vi "Main1.0.vi"() -> ()   [LabVIEW 2013]
panel:
  out "Log":string
  in  "Return":bool
  in  "DataCheckOut":bool
  in  "Setup":bool
  in  "EStop":bool
  in  "显示":enum32{"参数配置", "结果显示", "帮助"}(tab)
  in  "数据帧":T1
  in  "管理帧":T2
  in  "充电帧":T3
  in  "ECALL帧":T4
  in  "任意帧":T5
  in  "终端号码1":T6
  in  "终端号码2":T7
  in  "白名单号码":T8
  in  "黑名单号码":T9
  in  "ACC唤醒":T10
  in  "休眠":bool
  in  "CAN唤醒":bool
  in  "ACC唤醒":bool
  in  "短信唤醒":bool
  in  "电话唤醒":bool
  in  "ECALL唤醒":bool
  in  "长安测试配置":bool
  in  "江淮测试配置":bool
  in  "五菱测试配置":bool
  in  "长丰测试配置":bool
  in  "海马测试配置":bool
  in  "B+电压":u16(ring) items=["5.9V", "6.5V", "9V", "12V", "16V"]
  in  "休眠电流限值":dbl
  in  "工作电流限值":dbl
  in  "循环次数":dbl
  in  "间隔时间":dbl
  out "登录时间":dbl
  out "异常次数":dbl
  out "登录结果":bool
  out "TBOX状态":bool
  out "任意帧唤醒结果":T11
  out "无效短信唤醒结果":T11
  out "黑名单电话号码唤醒结果":T11
  out "白名单电话号码唤醒结果":T11
  out "指令短信唤醒结果":T11
  out "ECALL帧唤醒结果":T11
  out "充电帧唤醒结果":T11
  out "管理帧唤醒结果":T11
  out "数据帧唤醒结果":T11
  out "ACC唤醒结果":T11
  out "ACC异常计数":dbl caption="异常计数"
  out "管理帧异常计数":dbl caption="异常计数"
  out "数据帧异常计数":dbl caption="异常计数"
  out "充电帧异常计数":dbl caption="异常计数"
  out "ECALL帧异常计数":dbl caption="异常计数"
  out "任意帧异常计数":dbl caption="异常计数"
  out "指令短信异常计数":dbl caption="异常计数"
  out "无效短信异常计数":dbl caption="异常计数"
  out "白名单异常计数":dbl caption="异常计数"
  out "黑名单异常计数":dbl caption="异常计数"
  in  "Start":bool
  # "公用参数"
  # "测试流程选择"
  # "配置文件选择"
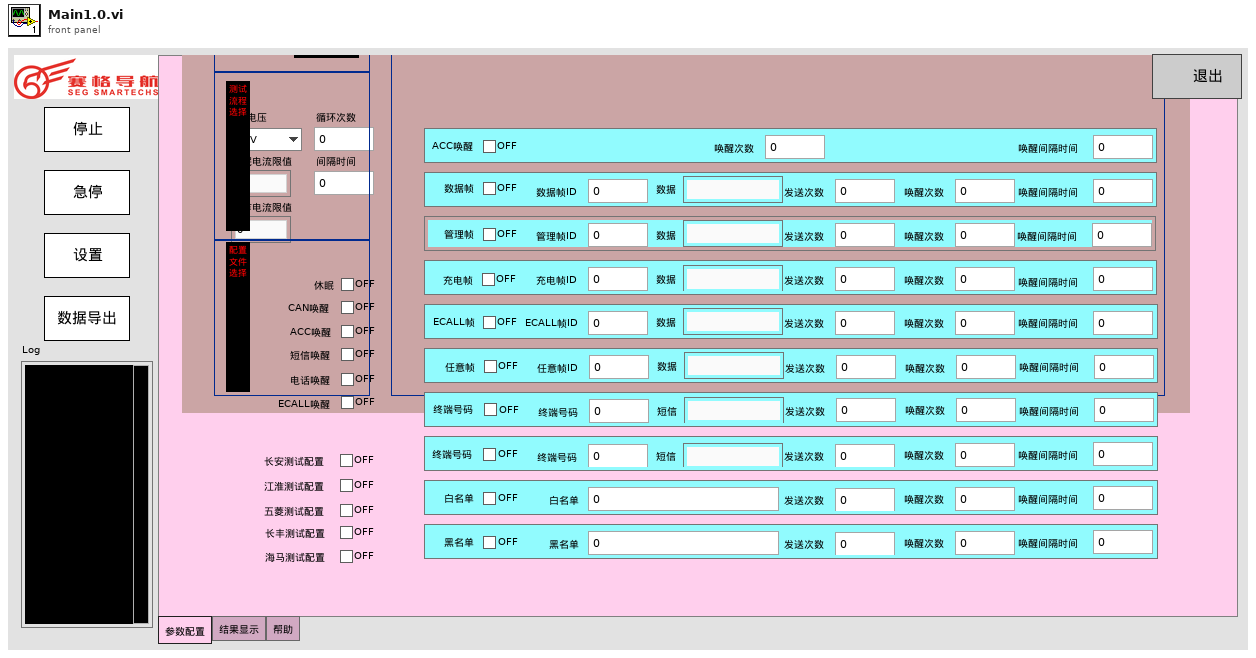
[diagram p1: front panel]
types:
  T1 = cluster{"数据帧":bool, "数据帧ID":dbl, "数据帧数据":string, "数据帧次数":dbl, "数据帧唤醒次数":dbl, "数据间隔时间":dbl}
  T2 = cluster{"管理帧":bool, "管理帧ID":dbl, "管理帧数据":string, "管理帧次数":dbl, "管理帧唤醒次数":dbl, "管理间隔时间":dbl}
  T3 = cluster{"充电帧":bool, "充电帧ID":dbl, "充电帧数据":string, "充电帧次数":dbl, "充电帧唤醒次数":dbl, "充电间隔时间":dbl}
  T4 = cluster{"ECALL帧":bool, "ECALL帧ID":dbl, "ECALL帧数据":string, "ECALL帧次数":dbl, "ECALL帧唤醒次数":dbl, "ECALL间隔时间":dbl}
  T5 = cluster{"任意帧ID":dbl, "任意帧数据":string, "任意帧次数":dbl, "任意帧唤醒次数":dbl, "任意间隔时间":dbl, "任意帧":bool}
  T6 = cluster{"终端号码1":dbl, "指令短信":string, "指令短信次数":dbl, "指令短信唤醒次数":dbl, "指令短信间隔时间":dbl, "终端号码":bool}
  T7 = cluster{"终端号码2":dbl, "无效短信":string, "无效短信次数":dbl, "无效短信唤醒次数":dbl, "无效短信间隔时间":dbl, "终端号码2 2":bool}
  T8 = cluster{"白名单":dbl, "白名单次数":dbl, "白名单唤醒次数":dbl, "白名单间隔时间":dbl, "白名单号码":bool}
  T9 = cluster{"黑名单":dbl, "黑名单次数":dbl, "黑名单唤醒次数":dbl, "黑名单间隔时间":dbl, "黑名单号码":bool}
  T10 = cluster{"ACC唤醒":bool, "ACC唤醒次数":dbl, "ACC间隔时间":dbl}
  T11 = cluster{"休眠电流":string, "工作电流":string, "唤醒结果":string, "登录状态":string}
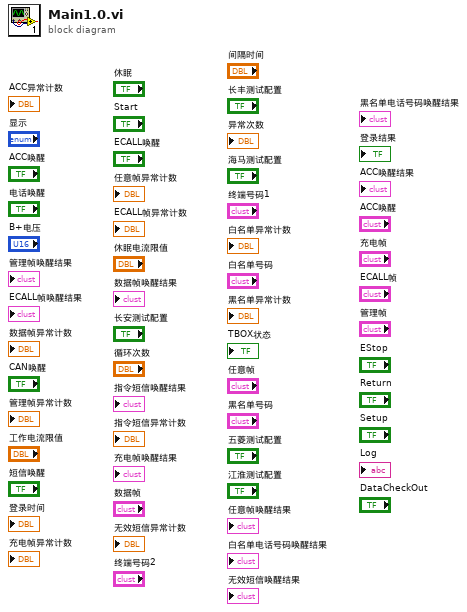
[diagram p0: block diagram]
diagram:
